vi "Write IO Task.vi"(8 "error in (no error)":errorcluster, 9 "IO Task":refnum<k21>, 10 "Task Name":string, 11 "Gantry in":refnum<class "Gantry.lvclass">) -> (0 "error out":errorcluster, 3 "Gantry out":refnum<class "Gantry.lvclass">)   [LabVIEW 2023, in "Gantry.lvclass"]
uses:
  Gantry.lvclass
  Gantry.lvclass/Gantry.ctl
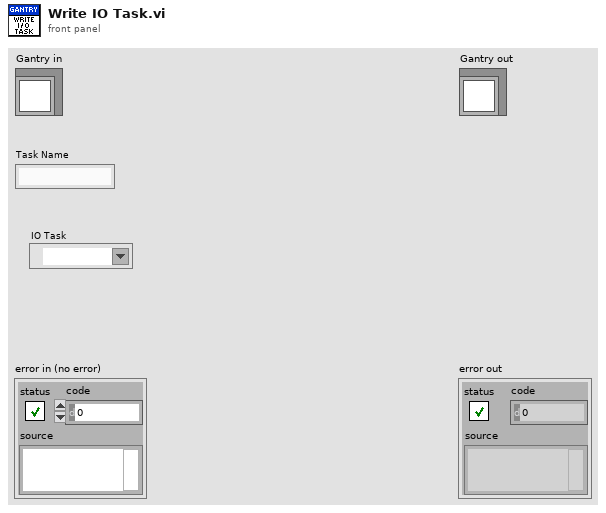
[diagram p1: front panel]
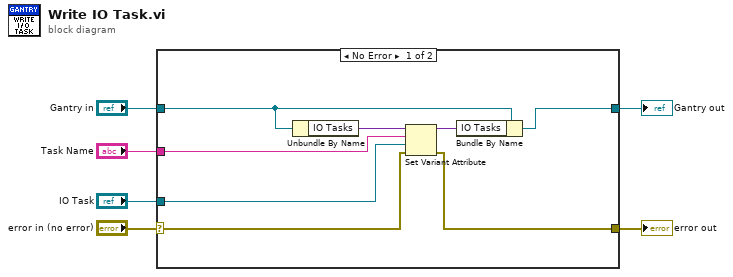
[diagram p0: block diagram]
diagram:
  n1 = case shown="No Error" "error in (no error)" {
    selector: "error in (no error)" -> [w11 w16]
    tunnel: [w8 w16] -> w5
    tunnel: [w7 w15] -> w3
    tunnel: "Gantry in" -> [w10 w15]
    tunnel: "Task Name" -> [w13 _]
    tunnel: "IO Task" -> [w12 _]
    frame No Error {
      n2 = Unbundle By Name(w10) -> ("IO Tasks"=w14:variant)
      n3 = Set Variant Attribute(Variant=w14, name=w13, value=w12, error in=w11) -> (Variant out=w9:variant, error out=w8:errorcluster)  [unwired: 1 out]
      n4 = Bundle By Name(cluster=w10, "IO Tasks"=w9) -> (w7:refnum<class "Gantry.lvclass">)
    }
    frame Error {
    }
  }
  "error out" <- w5
  "Gantry out" <- w3
